vi "ExSimpleRF.vi"() -> ()   [LabVIEW 2013]
uses:
  <vilib>/Utility/file.llb/Write To Spreadsheet File (DBL).vi
panel:
  in  "Save?":bool
  out "Waveform Graph":dbl[](graph)
  in  "Exposure":dbl=0.001 format="%.3f"
  in  "Close Compensation time ms 2":u32=8
  in  "Open Compensation time ms":u32=8
  in  "Temperature":dbl format="%.2f"
  out "error out":errorcluster
  in  "error in (no error)":errorcluster
  # "Note: for the Cascade and\nPhotonMax the open/close\n compensation should be 0"
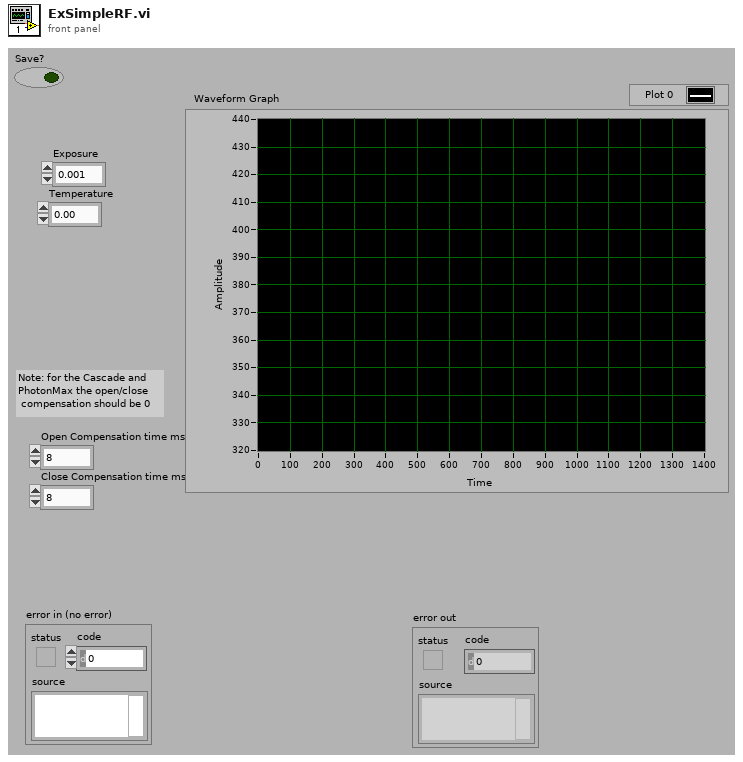
[diagram p1: front panel]
types:
  T1 = cluster{"Open Compensation time ms":u32, "Close Compensation time ms 2":u32}
  T2 = cluster{"Camera Handle":u32, "File Handle":u32, "Image Handle":u32}
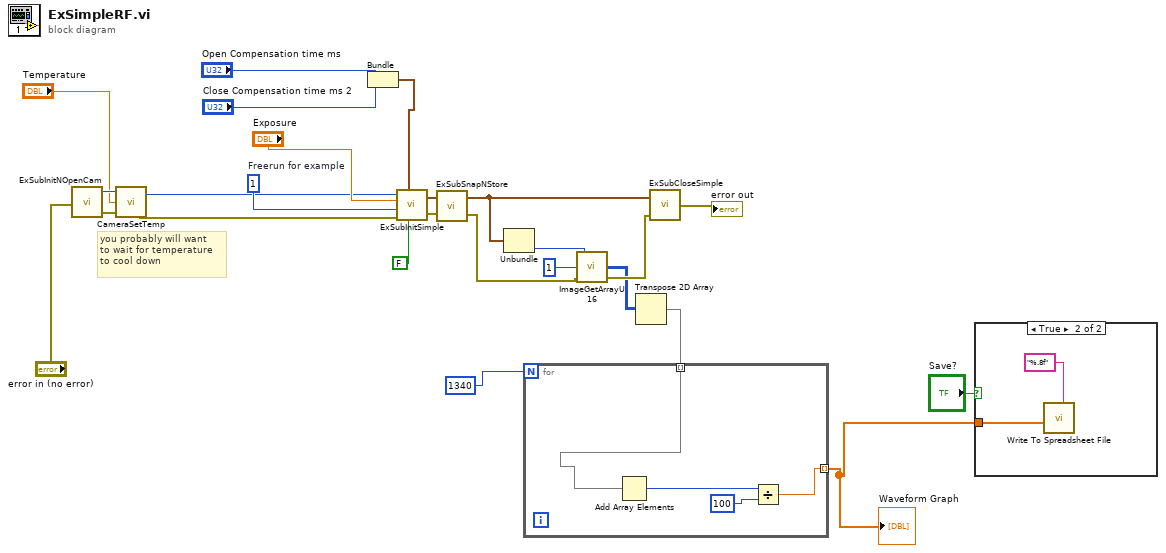
[diagram p0: block diagram]
diagram:
  w12 = 1  # Freerun for example
  # "you probably will want \nto wait for temperature \nto cool down"
  n1 = call "ExSubInitNOpenCam.vi"("error in (no error)"="error in (no error)") -> ("Camera Handle"=w23:u32, "error out"=w24:errorcluster)
  n2 = call <userlib>:"CameraSetTemp.vi"("error in (no error)"=w24, "Temperature"="Temperature", "Camera Handle"=w23) -> ("error out"=w18:errorcluster, "Camera Handle"=w11:u32)
  n3 = Bundle("Open Compensation time ms"="Open Compensation time ms", "Close Compensation time ms 2"="Close Compensation time ms 2") -> (w15:T1)  [unwired: 1 in]
  n4 = call "ExSubInitSimple.vi"("Intensifier"=FALSE, "Shutter Comp"=w15, "error in (no error)"=w18, "Triggering mode"=w12, "Exposure"="Exposure", "Camera Handle"=w11) -> ("error out"=w19:errorcluster, "Handles"=w20:cluster{"Camera":u32, "File":u32, "Image":u32})
  n5 = call "ExSubSnapNStore.vi"("error in (no error)"=w19, "Handle Cluster"=w20) -> ("error out"=w8:errorcluster, "Handle Cluster Out"=w10:T2)
  n6 = Unbundle(w10) -> ("Image Handle"=w9:u32)  [unwired: 2 out]
  n7 = call <userlib>:"ImageGetArrayU16.vi"("error in"=w8, "Z position"=1, "Image Handle"=w9) -> ("error out"=w7:errorcluster, "Array uint 16"=w5:u16[][])  [unwired: 1 out]
  n8 = Transpose 2D Array(2D array=w5) -> (transposed array=w3:u16[][])
  n9 = for {
    N: 1340 -> [_]
    tunnel: w3 -> [w29] mode=indexing
    tunnel: [w26] -> w1 mode=indexing
    n10 = Add Array Elements(numeric array=w29) -> (sum=w28:u16)
    n11 = Divide(x=w28, y=100) -> (x/y=w26:dbl)
  }
  "Waveform Graph" <- w1
  n12 = call "ExSubCloseSimple.vi"("error in (no error)"=w7, "Handles In"=w10) -> ("error out"=→"error out":errorcluster)
  n13 = case shown="True" "Save?" {
    tunnel: w1 -> [_ w31]
    frame False {
    }
    frame True {
      n14 = call-poly <vilib>:"Write To Spreadsheet File.vi"("format (%.3f)"="%.8f", "1D data"=w31) -> ()  [unwired: 6 in, 1 out]
    }
  }
